vi "Server_largefile.vi"() -> ()   [LabVIEW 2016, in "Sending_larger_data.lvlib"]
uses:
  Sending_larger_data.lvlib
  <vilib>/addons/zeromq/socket_type.ctl
  <vilib>/addons/zeromq/zmq_context.lvclass
  <vilib>/addons/zeromq/zmq_socket.lvclass
  <vilib>/addons/zeromq/zeromq.lvlib
  <vilib>/Analysis/NI_AALPro.lvlib
  <vilib>/Analysis/2dsp.llb/Power Spectrum (DBL).vi
panel:
  out "Power Spectrum":dbl[](graph)
  out "Signal Time domain":dbl[](graph)
  in  "stop?":bool
  out "loop":i32
  in  "endpoint":string="tcp://127.0.0.1:5555"
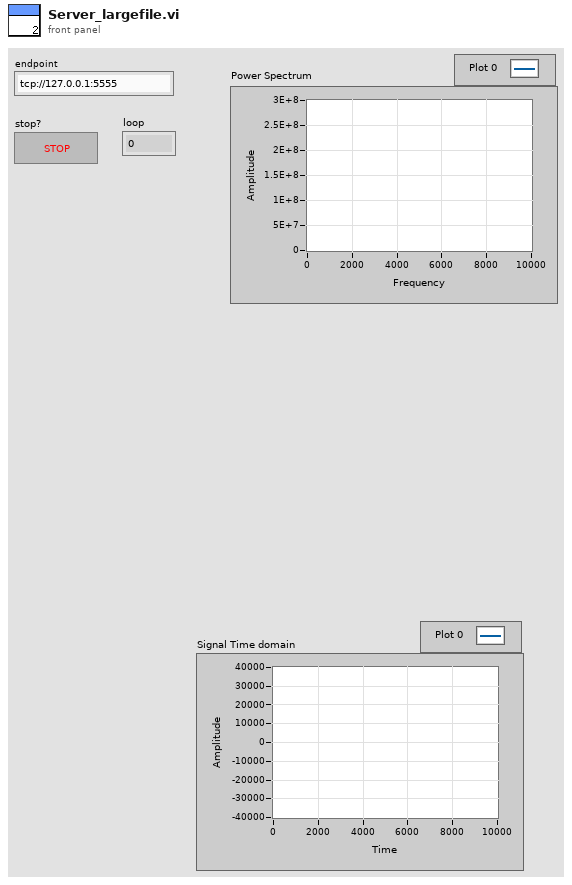
[diagram p1: front panel]
types:
  T1 = typedef "zeromq.lvlib/socket_type.ctl" = enum8{"ZMQ_PAIR", "ZMQ_PUB", "ZMQ_SUB", "ZMQ_REQ", "ZMQ_REP", "ZMQ_DEALER", "ZMQ_ROUTER", "ZMQ_PULL", "ZMQ_PUSH", "ZMQ_XPUB", "ZMQ_XSUB"}
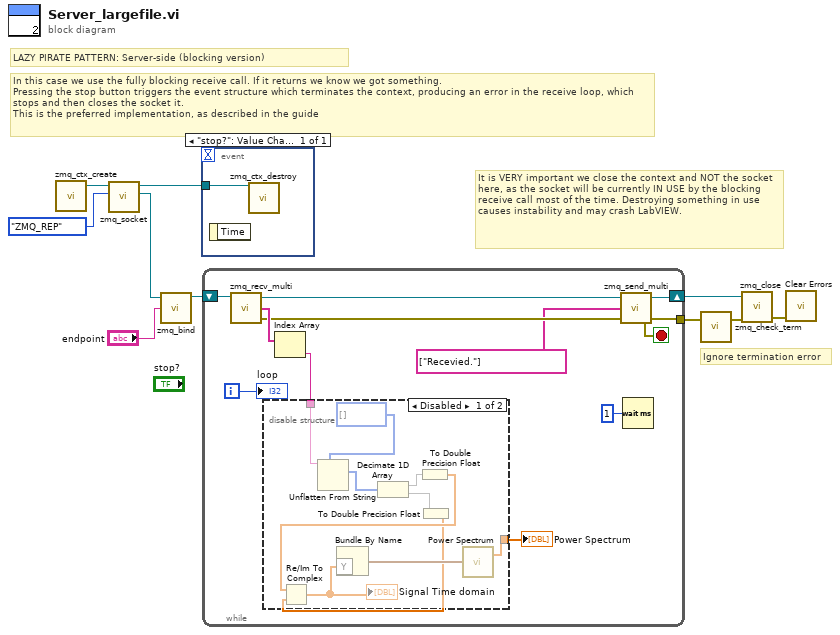
[diagram p0: block diagram]
diagram:
  # "Ignore termination error"
  # "It is VERY important we close the context and NOT the socket here, as the socket will be currently IN USE by the blocking receive call most of the time. Destroying something in use causes instability and may crash LabVIEW."
  # "In this case we use the fully blocking receive call. If it returns we know we got something.\nPressing the stop button triggers the event structure which terminates the context, producing an error in the receive loop, which stops and then closes the socket it.\nThis is the preferred implementation, as described in the guide"
  # "LAZY PIRATE PATTERN: Server-side (blocking version)"
  n1 = call <vilib>:"zmq_ctx_create.vi"() -> ("context out"=w6:refnum<class "zmq_context.lvclass">)  [unwired: 4 in, 1 out]
  n2 = call <vilib>:"zmq_socket.vi"("socket type"=socket_type."ZMQ_REP", "context in"=w6) -> ("socket out"=w5:refnum<class "zmq_socket.lvclass">, "context out"=w4:refnum<class "zmq_context.lvclass">)  [unwired: 3 in, 1 out]
  n3 = call <vilib>:"zmq_bind.vi"("endpoint"="endpoint", "socket in"=w5) -> ("socket out"=w9:refnum<class "zmq_socket.lvclass">)  [unwired: 2 in, 1 out]
  n4 = event shown="[0] \"stop?\": Value Change" {
    selector: _ -> [_]
    dyn-events: _ -> [_]
    timeout: _ -> [_]
    tunnel: w4 -> [w11]
    event "stop?": Value Change {
      n5 = event-data() -> ()  [unwired: 1 in, 1 out]
      n6 = call <vilib>:"zmq_ctx_destroy.vi"("context in"=w11) -> ()  [unwired: 4 in, 1 out]
    }
  }
  n7 = while {
    shift-right: [w19] -> w7
    shift-left: w9 -> [w22]
    tunnel: [w16] -> w2
    i -> [w18]
    stop <- w16 stop-if-true
    n8 = call <vilib>:"zmq_recv_multi.vi"("socket in"=w22) -> ("error out"=w17:errorcluster, "parts"=w20:string[], "socket out"=w21:refnum<class "zmq_socket.lvclass">)  [unwired: 2 in]
    n9 = Index Array(array=w20) -> (element=w15:string)  [unwired: 1 in]
    n10 = disable-structure shown="Disabled" {
      disable-tunnel: w15 -> [w32 _]
      disable-tunnel: [w23 _] -> w13
      frame Disabled {
        n11 = Unflatten From String(type=i16[] [], binary string=w32) -> (value=w30:i16[])  [unwired: 3 in, 2 out]
        n12 = Decimate 1D Array(w30) -> (w29:i16[], w28:i16[])
        n13 = To Double Precision Float(number=w29) -> (double precision float=w25:dbl[])
        n14 = To Double Precision Float(number=w28) -> (double precision float=w24:dbl[])
        n15 = Re/Im To Complex(1:w24, 2:w25) -> (0:w27:cdb[])
        "Signal Time domain" <- w27
        n16 = Bundle By Name("Y"=w27) -> (w26:waveform(cdb))  [unwired: 1 in]
        n17 = call-poly <vilib>:"Power Spectrum.vi"("X"=w26) -> ("Power Spectrum"=w23:dbl[])  [unwired: 1 out]
      }
      frame Enabled {
      }
    }
    "Power Spectrum" <- w13
    n18 = call <vilib>:"zmq_send_multi.vi"("error in"=w17, "parts"=string[] ["Recevied."], "socket in"=w21) -> ("error out"=w16:errorcluster, "socket out"=w19:refnum<class "zmq_socket.lvclass">)  [unwired: 1 in]
    n19 = Wait (ms)(milliseconds to wait=u32 1) -> ()  [unwired: 1 out]
    "loop" <- w18
  }
  n20 = call <vilib>:"zmq_check_term.vi"("error in"=w2) -> ("error out"=w1:errorcluster)  [unwired: 1 in, 1 out]
  n21 = call <vilib>:"zmq_close.vi"("error in"=w1, "socket"=w7) -> ("error out"=w3:errorcluster)  [unwired: 3 in]
  n22 = call <vilib>:"Clear Errors.vi"("error in (no error)"=w3) -> ()  [unwired: 5 in, 2 out]
